vi "GetSignalIndexByName.vi"(10 "Signal Name":string, 11 "Signal Array In":T1[](array[typedef])) -> (2 "Signal Found":bool, 3 "Index Out":u32)   [LabVIEW 2016]
uses:
  Ctrl_Signal.ctl
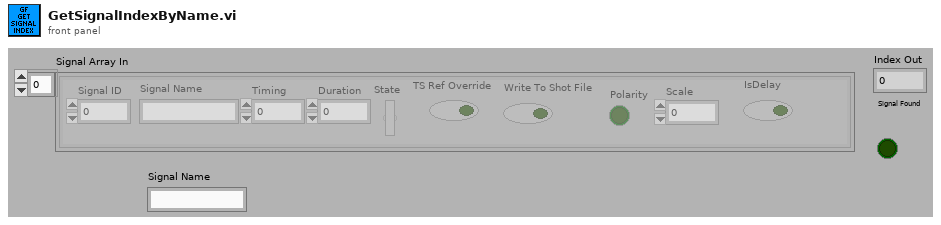
[diagram p1: front panel]
types:
  T1 = typedef "Ctrl_Signal.ctl" = cluster{"Signal Name":string, "Timing":dbl, "Duration":dbl, "State":bool, "TS Ref Override":bool, "Write To Shot File":bool, "Polarity":bool, "Signal ID":dbl, "Scale":dbl, "IsDelay":bool}
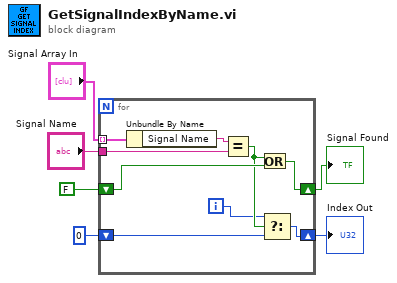
[diagram p0: block diagram]
diagram:
  n1 = for {
    tunnel: "Signal Array In" -> [w15] mode=indexing
    tunnel: "Signal Name" -> [w13]
    shift-right: [w11] -> w3
    shift-left: FALSE -> [w12]
    shift-right: [w8] -> w1
    shift-left: u32 0 ("Index Out") -> [w9]
    i -> [w7]
    n2 = Unbundle By Name(w15) -> ("Signal Name"=w14:string)
    n3 = Equal?(x=w14, y=w13) -> (x = y?=w10:bool)
    n4 = Or(x=w10, y=w12) -> (x .or. y?=w11:bool)
    n5 = Select(t=w7, s=w10, f=w9) -> (s? t:f=w8:u32)
  }
  "Signal Found" <- w3
  "Index Out" <- w1
